vi "roboRIO v1.0 Scaling Constants Table.vi"() -> ()   [LabVIEW 2021]
panel:
  in  "roboRIO v1.0 Scaling Constant Table":string="Not Connected;0;0;0\nB/AI0;1220703;0;0\nB/AI1;1220703;0;0\nB/AI2;1220703;0;0\nB/AI3;1220703;0;0\nAI/AI0;1220703;0;0\nAI/AI1;1220703;0;0\nAI/AI2;1220703;0;0\nAI/AI3;1220703;0;0\nB/AO0;1220703;0;0\nB/AO1;1220703;0;0\nONBOARD/ACC;256\nB/AI0 (Interrupt);1220703;0;0\nB/AI1 (Interrupt);1220703;0;0"
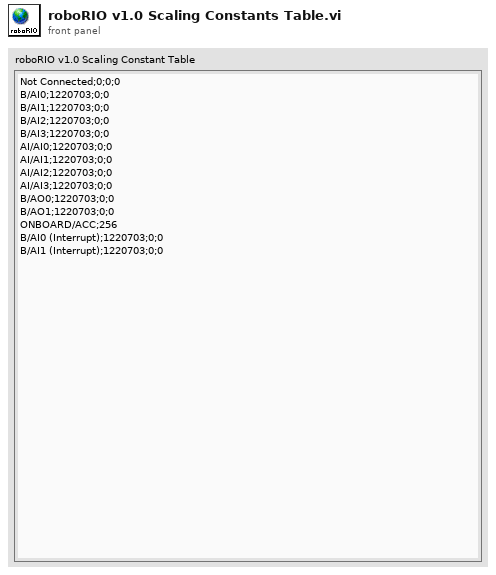
[diagram p1: front panel]
diagram:
